vi "MSEncoder Case-9-UpdIGVolts.vi"(8 "error in (no error)":errorcluster, 9 "ParamValIn":variant, 11 "MSEncoder in":refnum<class "MSEncoder.lvclass">) -> (0 "error out":errorcluster, 3 "MSEncoder out":refnum<class "MSEncoder.lvclass">)   [LabVIEW 2018, in "MSEncoder.lvclass"]
uses:
  MSEncoder.lvclass
  Ctl/MSEditorParam updIGVolts.ctl
  MSEncoder.lvclass/MSEncoder.ctl
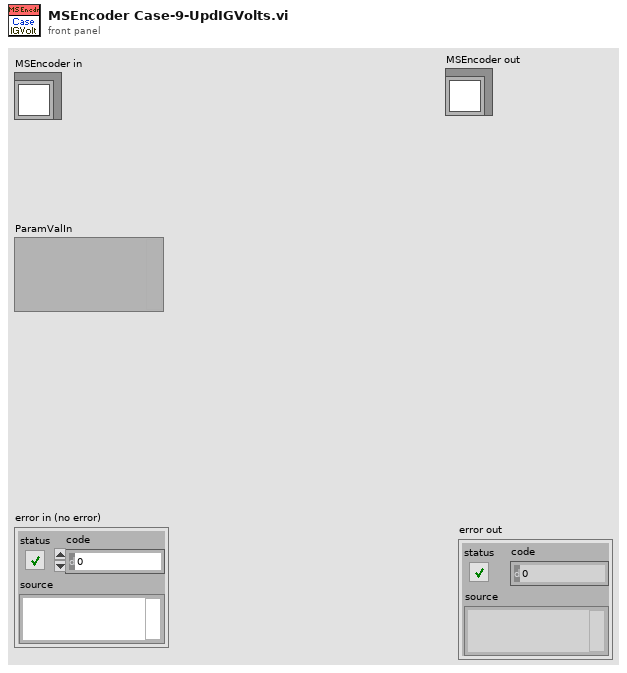
[diagram p1: front panel]
types:
  T1 = typedef "MSEditorParam updIGVolts.ctl" = cluster{"onVolt":dbl, "offVolt":dbl}
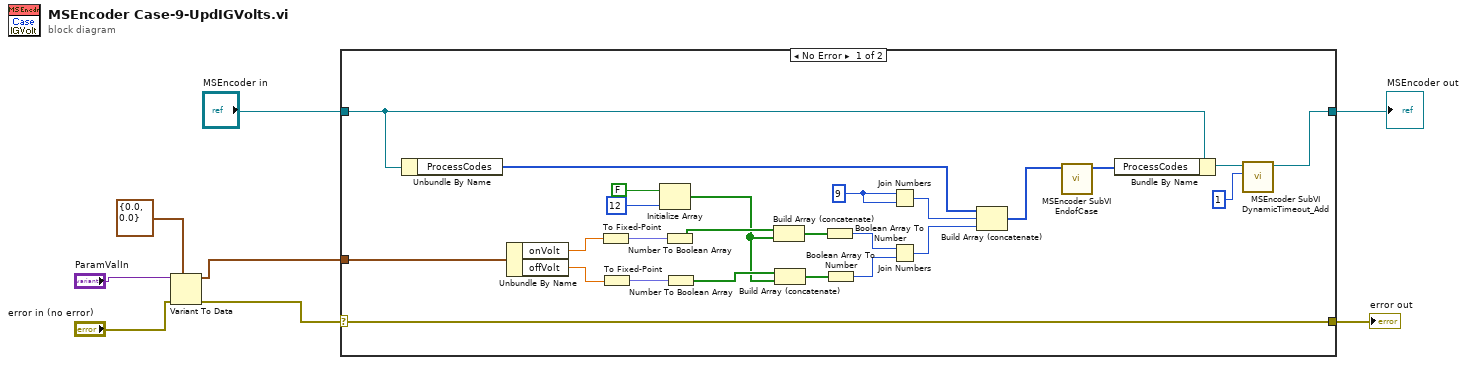
[diagram p0: block diagram]
diagram:
  n1 = Variant To Data(error in="error in (no error)", type=T1 {"onVolt"=0.0, "offVolt"=0.0} ("ParamValueType"), Variant="ParamValIn") -> (data=w3:T1, error out=w2:errorcluster)
  n2 = case shown="No Error" w2 {
    selector: w2 -> [w13 w35]
    tunnel: "MSEncoder in" -> [w32 w34]
    tunnel: [w13 w35] -> w8
    tunnel: [w10 w34] -> w6
    tunnel: w3 -> [w12 _]
    frame No Error {
      w30 = u32 9
      n3 = Unbundle By Name(w32) -> ("ProcessCodes"=w33:u64[])
      n4 = Unbundle By Name(w12) -> ("onVolt"=w15:dbl, "offVolt"=w14:dbl)
      n5 = To Fixed-Point(number=w15) -> (fixed-point=w27:fxp<+/-,20,5>)  [unwired: 1 in]
      n6 = To Fixed-Point(number=w14) -> (fixed-point=w26:fxp<+/-,20,5>)  [unwired: 1 in]
      n7 = Initialize Array(FALSE, 12 ("dimension size")) -> (w21:bool[])
      n8 = Number To Boolean Array(number=w27) -> (Boolean array=w23:bool[])
      n9 = Number To Boolean Array(number=w26) -> (Boolean array=w22:bool[])
      n10 = Build Array (concatenate)(w23, w21) -> (w20:bool[])
      n11 = Build Array (concatenate)(w22, w21) -> (w19:bool[])
      n12 = Boolean Array To Number(Boolean array=w20) -> (number=w17:u32)
      n13 = Boolean Array To Number(Boolean array=w19) -> (number=w18:u32)
      n14 = Join Numbers(hi=w30, lo=w30) -> ((hi.lo)=w29:u64)
      n15 = Join Numbers(hi=w17, lo=w18) -> ((hi.lo)=w28:u64)
      n16 = Build Array (concatenate)(w33, w29, w28) -> (w16:u64[])
      n17 = call "MSEncoder SubVI EndofCase.vi"("Case codes"=w16) -> ("Case codes with end"=w31:u64[])  [unwired: 9 in, 1 out]
      n18 = Bundle By Name(cluster=w32, "ProcessCodes"=w31) -> (w11:refnum<class "MSEncoder.lvclass">)
      n19 = call "MSEncoder SubVI DynamicTimeout_Add.vi"("Timeout_ms"=1, "MSEncoder"=w11) -> ("MSEncoder"=w10:refnum<class "MSEncoder.lvclass">)  [unwired: 8 in, 1 out]
    }
    frame Error {
    }
  }
  "error out" <- w8
  "MSEncoder out" <- w6
